vi "convert seconds to h min string.vi"(1 "time duration (seconds)":dbl format="%.2f seconds") -> (0 "running time string":string)   [LabVIEW 2020, in "main.lvlib"]
uses:
  main.lvlib
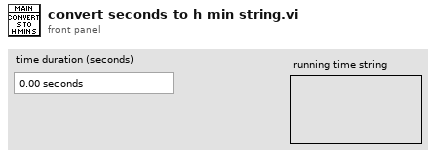
[diagram p1: front panel]
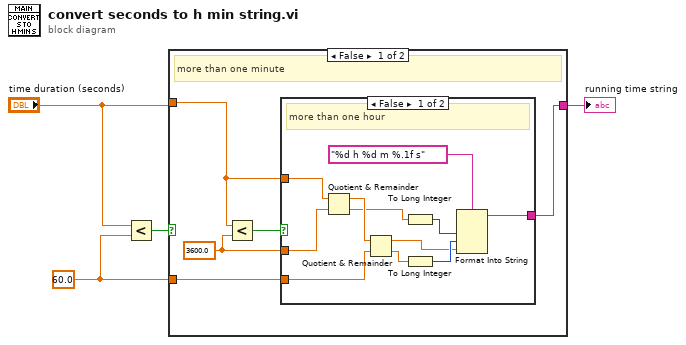
[diagram p0: block diagram]
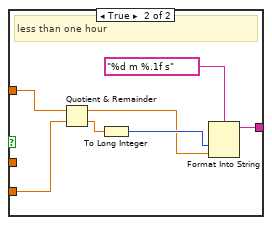
[diagram p2: hidden frame]
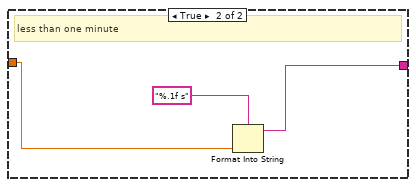
[diagram p3: hidden frame]
diagram:
  w1 = 60.0 ("y")
  n1 = Less?(x="time duration (seconds)", y=w1) -> (x < y?=w2:bool)
  n2 = case shown="False" w2 {
    tunnel: "time duration (seconds)" -> [w8 w29]
    tunnel: [w6 w28] -> w4
    tunnel: w1 -> [w7 _]
    frame False {
      w5 = 3600.0 ("y")
      # "more than one minute"
      n3 = Less?(x=w8, y=w5) -> (x < y?=w9:bool)
      n4 = case shown="False" w9 {
        tunnel: w8 -> [w20 w26]
        tunnel: w7 -> [w15 w25]
        tunnel: [w10 w21] -> w6
        tunnel: w5 -> [w19 _]
        frame False {
          # "more than one hour"
          n5 = Quotient & Remainder(x=w20, y=w19) -> (x-y*floor(x/y)=w16:dbl, floor(x/y)=w14:dbl)
          n6 = Quotient & Remainder(x=w16, y=w15) -> (x-y*floor(x/y)=w11:dbl, floor(x/y)=w17:dbl)
          n7 = To Long Integer(number=w14) -> (32bit integer=w13:i32)
          n8 = To Long Integer(number=w17) -> (32bit integer=w12:i32)
          n9 = Format Into String(format string="%d h %d m %.1f s", w13, w12, w11) -> (resulting string=w10:string)  [unwired: 2 in, 1 out]
        }
        frame True {
          # "less than one hour"
          n10 = Quotient & Remainder(x=w26, y=w25) -> (x-y*floor(x/y)=w22:dbl, floor(x/y)=w24:dbl)
          n11 = To Long Integer(number=w24) -> (32bit integer=w23:i32)
          n12 = Format Into String(format string="%d m %.1f s", w23, w22) -> (resulting string=w21:string)  [unwired: 2 in, 1 out]
        }
      }
    }
    frame True {
      # "less than one minute"
      n13 = Format Into String(format string="%.1f s", w29) -> (resulting string=w28:string)  [unwired: 2 in, 1 out]
    }
  }
  "running time string" <- w4
